vi "SubModule Read Data.vi"(8 "error in (no error)":errorcluster, 11 "Canon in":refnum<class "Canon.lvclass">) -> (0 "error out":errorcluster, 1 "Data":string[](array[string]), 3 "Canon out":refnum<class "Canon.lvclass">)   [LabVIEW 2021, in "Canon.lvclass"]
uses:
  Canon.lvclass
  C:/Projects/InstrPanel/Classes/Camera/Camera.lvclass
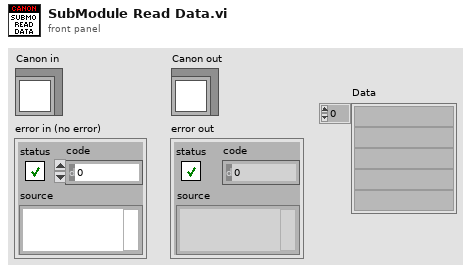
[diagram p1: front panel]
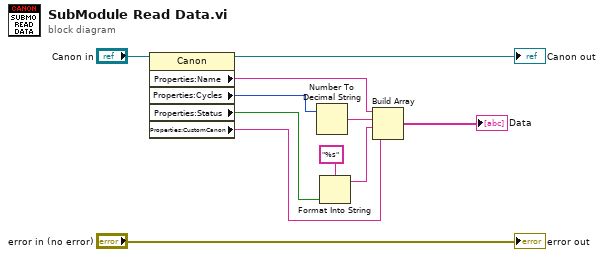
[diagram p0: block diagram]
diagram:
  n1 = property class="Canon"(reference="Canon in") -> (reference out=→"Canon out":refnum<class "Canon.lvclass">, "Properties:Name"=w6:string, "Properties:Cycles"=w8:i32, "Properties:Status"=w7:bool, "Properties:CustomCanon"=w3:string)  [unwired: 1 in, 1 out]
  n2 = Number To Decimal String(number=w8) -> (decimal integer string=w5:string)  [unwired: 1 in]
  n3 = Format Into String(format string="%s", w7) -> (resulting string=w4:string)  [unwired: 2 in, 1 out]
  n4 = Build Array(w6, w5, w4, w3) -> (→"Data":string[])
  "error out" <- "error in (no error)"
